vi "Write NI_API_ConnectionRef.vi"(8 "error in (no error)":errorcluster, 10 "reference":T1, 11 "NI_DB_API in":refnum<class "NI_DB_API.lvclass">) -> (0 "error out":errorcluster, 3 "NI_DB_API out":refnum<class "NI_DB_API.lvclass">)   [LabVIEW 2021, in "NI_DB_API.lvclass"]
uses:
  <userlib>/John_Lib/DataBase/NI_DB_API/NI_DB_API.lvclass
  <userlib>/John_Lib/DataBase/NI_DB_API/NI_DB_API.lvclass/NI_DB_API.ctl
  <vilib>/addons/database/Connection.llb/Conn ObjectReference.ctl
  <vilib>/addons/database/NI_Database_API.lvlib
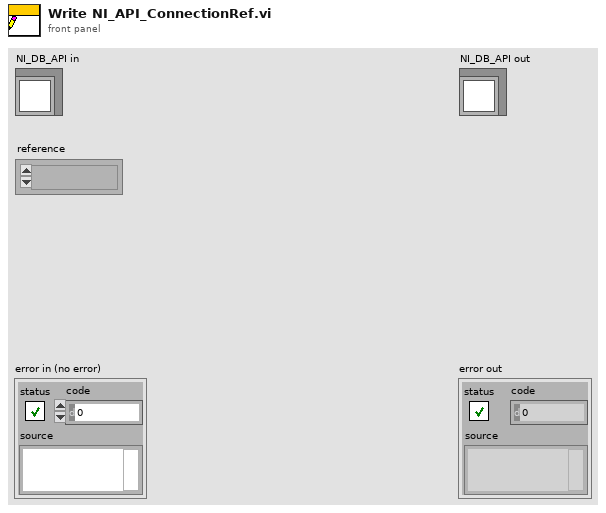
[diagram p1: front panel]
types:
  T1 = typedef "NI_Database_API.lvlib/Conn ObjectReference.ctl" = refnum<k1>
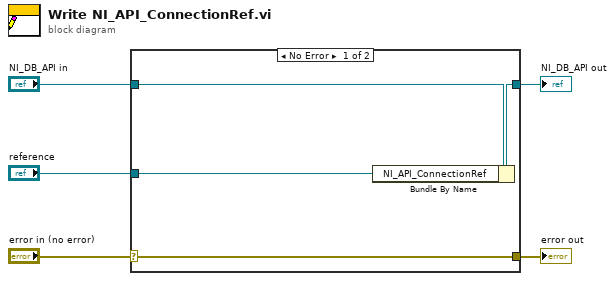
[diagram p0: block diagram]
diagram:
  n1 = case shown="No Error" "error in (no error)" {
    selector: "error in (no error)" -> [w9 w10]
    tunnel: [w9 w10] -> w4
    tunnel: [w7 w11] -> w2
    tunnel: "NI_DB_API in" -> [w8 w11]
    tunnel: "reference" -> [w6 _]
    frame No Error {
      n2 = Bundle By Name(cluster=w8, "NI_API_ConnectionRef"=w6) -> (w7:refnum<class "NI_DB_API.lvclass">)
    }
    frame Error {
    }
  }
  "error out" <- w4
  "NI_DB_API out" <- w2
